vi "Create Readings Table_Beltwatch.vi"() -> ()   [LabVIEW 2017, in "SQlkite Template.lvlib"]
uses:
  SQlkite Template.lvlib
  Common64/Database/SQ Lite/SQ Lite Cluster Action.ctl
panel:
  out "error out":errorcluster
  in  "Pre String":string="DROP TABLE IF EXISTS readings;\n\n\nCREATE TABLE readings (\n  db_id INTEGER PRIMARY KEY AUTOINCREMENT, \ndb_event_id INTEGER\n\n"
  in  "Readingse":T1[](array[typedef])=[{"Include"=TRUE, "Name"="Reading #", "SQLite3 type"=enum."SQLITE_INTEGER"}, {"Include"=TRUE, "Name"="Readings", "SQLite3 type"=enum."SQLITE3_TEXT"}, {"Include"=TRUE, "Name"="Reading Name", "SQLite3 type"=enum."SQLITE3_TEXT"}, {"Include"=TRUE, "Name"="Type", "SQLite3 type"=enum."SQLITE_INTEGER"}, {"Include"=TRUE, "Name"="Alarm priority", "SQLite3 type"=enum."SQLITE_INTEGER"}, {"Include"=TRUE, "Name"="Display precision", "SQLite3 type"=enum."undefined type (0)"}]
  out "?":errorcluster
  out "String":string
  out "SQLite3 type":T2(ring)
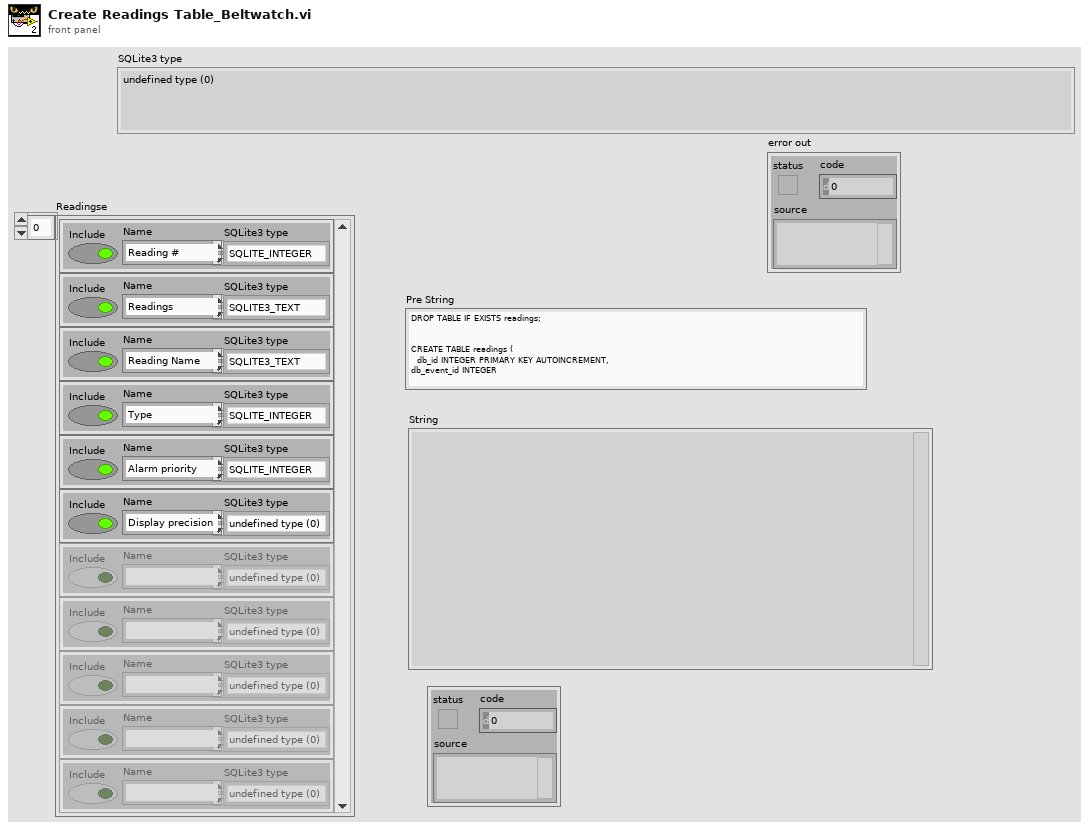
[diagram p1: front panel]
types:
  T1 = typedef "SQlkite Template.lvlib/SQ Lite Cluster Action.ctl" = cluster{"Include":bool, "Name":string, "SQLite3 type":enum32{"undefined type (0)", "SQLITE_INTEGER", "SQLITE_FLOAT", "SQLITE3_TEXT", "SQLITE_BLOB", "SQLITE_NULL", "undefined type"}}
  T2 = enum32{"undefined type (0)", "SQLITE_INTEGER", "SQLITE_FLOAT", "SQLITE3_TEXT", "SQLITE_BLOB", "SQLITE_NULL", "undefined type"}
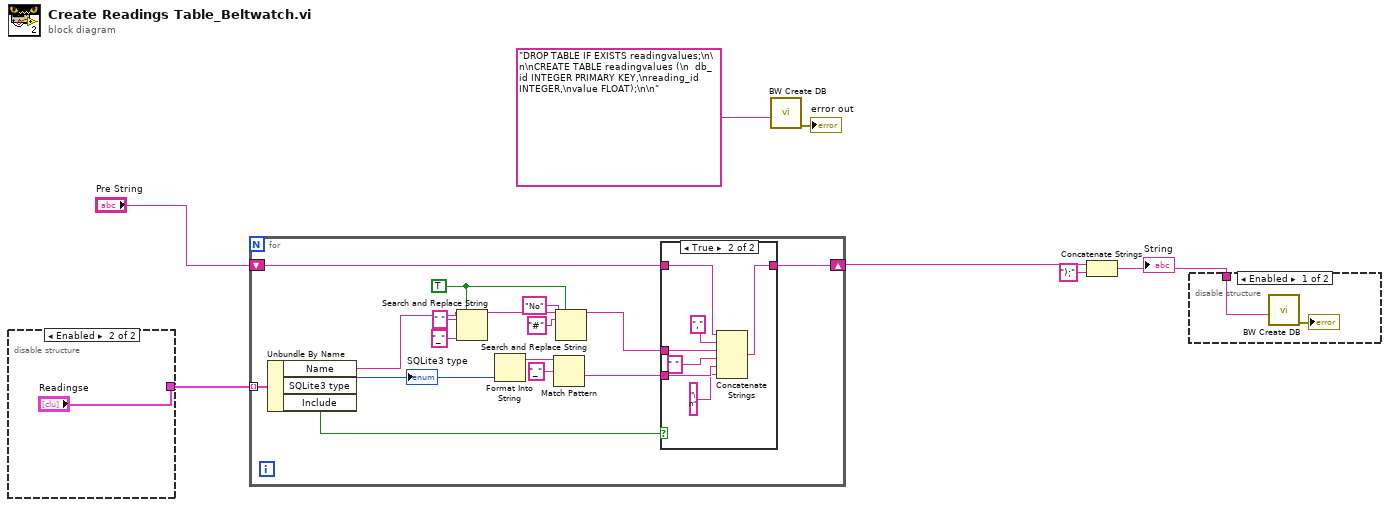
[diagram p0: block diagram]
diagram:
  n1 = disable-structure shown="Enabled" {
    disable-tunnel: [w8 "Readingse"] -> w6
    frame Disabled {
    }
    frame Enabled {
    }
  }
  n2 = for {
    shift-right: [w18] -> w5
    shift-left: "Pre String" -> [w25]
    tunnel: w6 -> [w24] mode=indexing
    w14 = TRUE ("replace all? (F)")
    n3 = Unbundle By Name(w24) -> ("Name"=w17:string, "SQLite3 type"=w22:T2, "Include"=w23:bool)
    "SQLite3 type" <- w22
    n4 = Search and Replace String(replace all?=w14, input string=w17, search string=" ", replace string="_" ("replace string (\"\")")) -> (result string=w13:string)  [unwired: 4 in, 3 out]
    n5 = Format Into String(w22) -> (resulting string=w21:string)  [unwired: 3 in, 1 out]
    n6 = Match Pattern(string=w21, regular expression="_") -> (after substring=w19:string)  [unwired: 1 in, 3 out]
    n7 = Search and Replace String(replace all?=w14, input string=w13, search string="#" ("replace string (\"\")"), replace string="No" ("replace string (\"\")")) -> (result string=w10:string)  [unwired: 4 in, 3 out]
    n8 = case shown="True" w23 {
      tunnel: w25 -> [w26 w28]
      tunnel: w10 -> [_ w33]
      tunnel: w19 -> [_ w31]
      tunnel: [w26 w30] -> w18
      frame False {
      }
      frame True {
        n9 = Concatenate Strings(w28, "," ("string"), w33, " " ("string"), w31, "\n" ("string")) -> (w30:string)
      }
    }
  }
  n10 = call "BW Create DB.vi"("String"="DROP TABLE IF EXISTS readingvalues;\n\n\nCREATE TABLE readingvalues (\n  db_id INTEGER PRIMARY KEY,\nreading_id INTEGER,\nvalue FLOAT);\n\n" ("Pre String")) -> ("error out"=→"error out":errorcluster)  [unwired: 10 in]
  n11 = Concatenate Strings(w5, ");" ("string")) -> (w3:string)
  "String" <- w3
  n12 = disable-structure shown="Enabled" {
    disable-tunnel: w3 -> [w35 _]
    frame Enabled {
      n13 = call "BW Create DB.vi"("String"=w35) -> ("error out"=→"?":errorcluster)  [unwired: 10 in]
    }
    frame Disabled {
    }
  }
